vi "Wait.vi"(8 "error in (no error)":errorcluster, 10 "Params":variant, 11 "NI DAQmx Base in":refnum<class "NI DAQmx Base.lvclass">) -> (0 "error out":errorcluster, 3 "NI DAQmx Base out":refnum<class "NI DAQmx Base.lvclass">)   [LabVIEW 2020, in "NI DAQmx.lvlib" / "NI DAQmx Base.lvclass"]
uses:
  NI DAQmx Base.lvclass
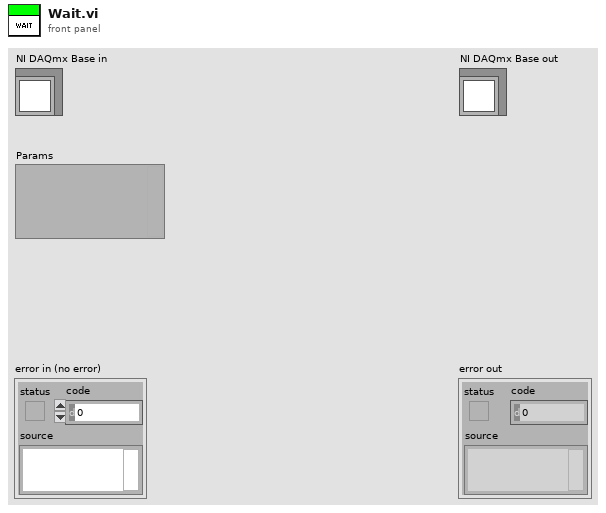
[diagram p1: front panel]
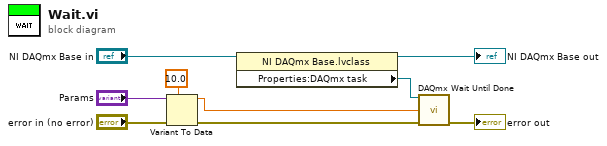
[diagram p0: block diagram]
diagram:
  n1 = Variant To Data(error in="error in (no error)", type=10.0 ("timeout (sec)"), Variant="Params") -> (data=w1:dbl, error out=w2:errorcluster)
  n2 = property class="NI DAQmx Base.lvclass"(reference="NI DAQmx Base in") -> (reference out=→"NI DAQmx Base out":refnum<class "NI DAQmx Base.lvclass">, "Properties:DAQmx task"=w7:refnum<k21>)  [unwired: 1 in, 1 out]
  n3 = call <vilib>:"DAQmx Wait Until Done.vi"("task/channels in"=w7, "timeout (sec)"=w1, "error in"=w2) -> ("error out"=→"error out":errorcluster)  [unwired: 11 in, 1 out]
